vi "datalog.vi"(9 "Incorrect_data":dbl, 10 "Correct_data":dbl, 11 "Total_data":dbl) -> ()   [LabVIEW 2017]
uses:
  <vilib>/Utility/file.llb/Write Delimited Spreadsheet (string).vi
  <vilib>/Utility/file.llb/Write Delimited Spreadsheet (DBL).vi
panel:
  out "Array":string[](array[string])
  in  "stop":bool
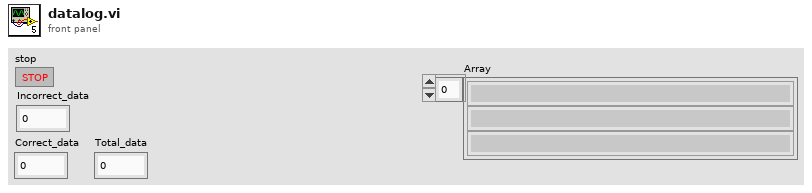
[diagram p1: front panel]
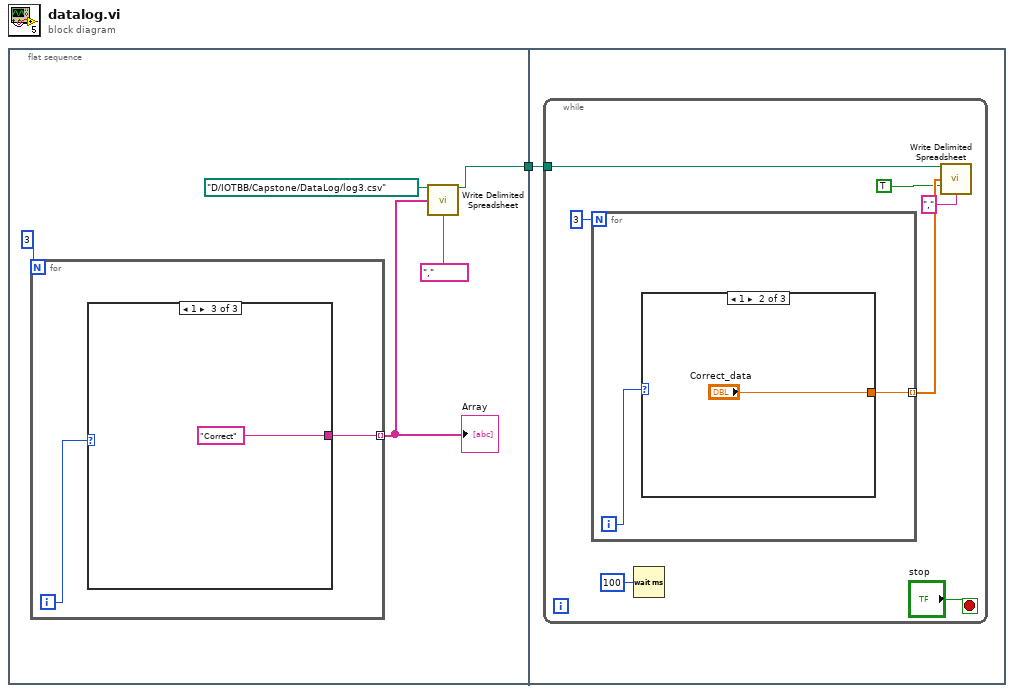
[diagram p0: block diagram]
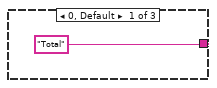
[diagram p2: hidden frame]
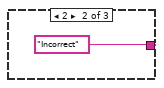
[diagram p3: hidden frame]
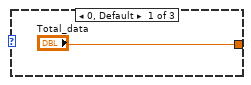
[diagram p4: hidden frame]
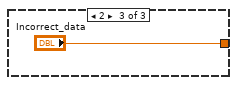
[diagram p5: hidden frame]
diagram:
  n1 = flat-sequence {
    tunnel: [w3] -> w1
    tunnel: w1 -> [w12]
    frame #0 {
      n2 = for {
        N: 3 -> [_]
        tunnel: [w7] -> w5 mode=indexing
        i -> [w8]
        n3 = case shown="1" w8 {
          tunnel: ["Total" "Incorrect" "Correct"] -> w7
          frame 0, Default {
          }
          frame 2 {
          }
          frame 1 {
          }
        }
      }
      "Array" <- w5
      n4 = call-poly <vilib>:"Write Delimited Spreadsheet.vi"("file path (dialog if empty)"=path "D:/IOTBB/Capstone/DataLog/log3.csv", "1D data"=w5, "delimiter (\\t)"="," ("delimiter (\\t)")) -> ("new file path (Not A Path if cancelled)"=w3:path)  [unwired: 11 in, 1 out]
    }
    frame #1 {
      n5 = while {
        tunnel: w12 -> [w17]
        stop <- "stop" stop-if-true
        n6 = for {
          N: 3 -> [_]
          tunnel: [w20] -> w16 mode=indexing
          i -> [w21]
          n7 = case shown="1" w21 {
            tunnel: ["Total_data" "Correct_data" "Incorrect_data"] -> w20
            frame 0, Default {
            }
            frame 1 {
            }
            frame 2 {
            }
          }
        }
        n8 = Wait (ms)(milliseconds to wait=u32 100) -> ()  [unwired: 1 out]
        n9 = call-poly <vilib>:"Write Delimited Spreadsheet.vi"("file path (dialog if empty)"=w17, "1D data"=w16, "append to file? (new file:F)"=TRUE, "delimiter (\\t)"="," ("delimiter (\\t)")) -> ()  [unwired: 10 in, 2 out]
      }
    }
  }
